vi "Intake Problem Fix.vi"(1 "Operator Intake Modified":T3, 2 "Operator Intake Original":T3) -> (0 "Operator Intake Fixed":T3)   [LabVIEW 2013]
uses:
  <vilib>/Rock Robotics/WPI/Relay/WPI_RelayValue.ctl
  <vilib>/Rock Robotics/WPI/Solenoid/WPI_SolenoidValue.ctl
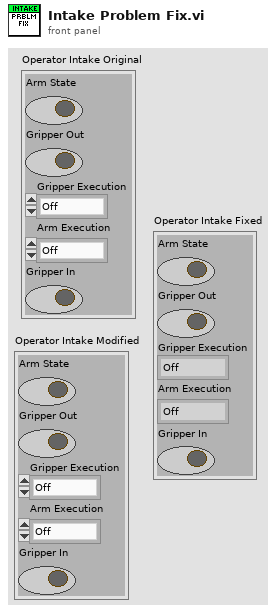
[diagram p1: front panel]
types:
  T1 = typedef "WPI_RelayValue.ctl" = enum16{"Off", "On", "Forward", "Reverse"}
  T2 = typedef "WPI_SolenoidValue.ctl" = enum16{"Off", "On", "Forward", "Reverse"}
  T3 = cluster{"Arm State":bool, "Gripper Out":bool, "Gripper Execution":T1, "Arm Execution":T2, "Gripper In":bool}
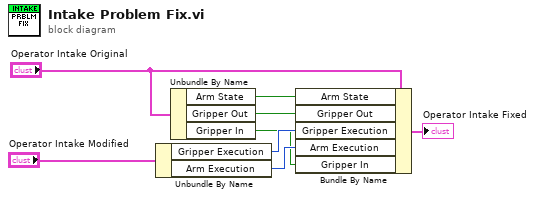
[diagram p0: block diagram]
diagram:
  n1 = Unbundle By Name("Operator Intake Modified") -> ("Gripper Execution"=w3:T1, "Arm Execution"=w2:T2)
  n2 = Unbundle By Name("Operator Intake Original") -> ("Arm State"=w8:bool, "Gripper Out"=w7:bool, "Gripper In"=w1:bool)
  n3 = Bundle By Name(cluster="Operator Intake Original", "Arm State"=w8, "Gripper Out"=w7, "Gripper Execution"=w3, "Arm Execution"=w2, "Gripper In"=w1) -> (→"Operator Intake Fixed":T3)
